vi "Read_AutoGeneralInput.vi"(8 "error in (no error)":errorcluster, 11 "AutoSubsystem in":refnum<class "AutoSubroutine.lvclass">) -> (0 "error out":errorcluster, 2 "GeneralAutoInput":T1, 3 "AutoSubsystem out":refnum<class "AutoSubroutine.lvclass">)   [LabVIEW 2017, in "AutoSubroutine.lvclass"]
uses:
  AutoSubroutine.lvclass
  AutoInput.ctl
  AutoSubroutine.lvclass/AutoSubroutine.ctl
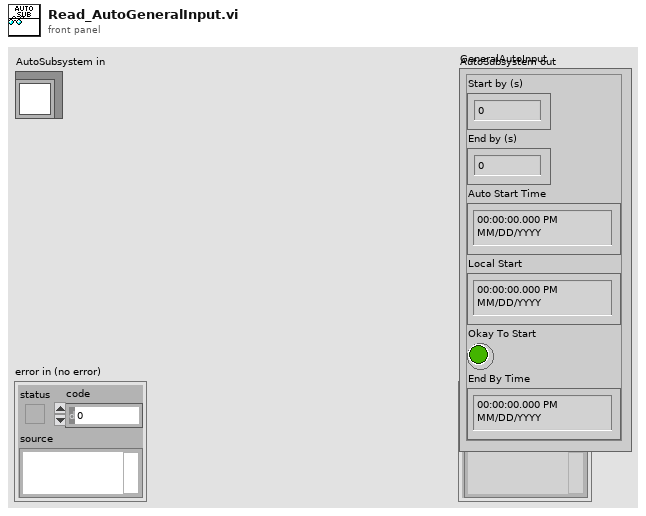
[diagram p1: front panel]
types:
  T1 = typedef "AutoSubroutine.lvclass/AutoInput.ctl" = cluster{"Start by (s)":dbl, "End by (s)":dbl, "Auto Start Time":timestamp, "Local Start":timestamp, "Okay To Start":bool, "End By Time":timestamp}
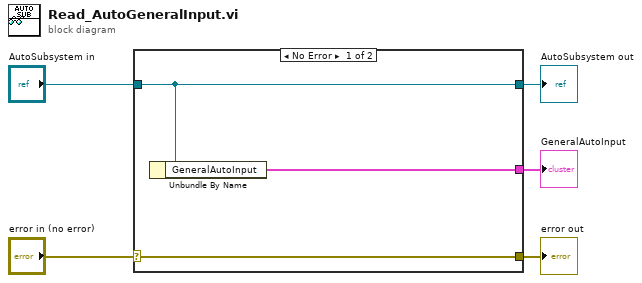
[diagram p0: block diagram]
diagram:
  n1 = case shown="No Error" "error in (no error)" {
    selector: "error in (no error)" -> [w8 w9]
    tunnel: [w8 w9] -> w4
    tunnel: [w7 w10] -> w2
    tunnel: "AutoSubsystem in" -> [w7 w10]
    tunnel: [w6 _] -> w1
    frame No Error {
      n2 = Unbundle By Name(w7) -> ("GeneralAutoInput"=w6:T1)
    }
    frame Error {
    }
  }
  "error out" <- w4
  "AutoSubsystem out" <- w2
  "GeneralAutoInput" <- w1
